vi "TEST_ASIC_MAJ_(3RD)_NEW.vi"(4 "Voltages comprobation":dbl[](array[numeric])=[0.05, 0.1, 0.2, 0.5, 0.8], 7 "Serial number":string="SN_023", 8 "error in":errorcluster, 9 "Cycles Burst":i32=10000, 10 "Channels":i32[](array[numeric])=[0, 1, 2, 3, 4, 5, 6], 11 "Instrument VISA in":T1={"AWG VISA"="generadorpulsos", "Oscilloscope  VISA "="Oscilloscope", "Integration Board IP"="172.16.7.43", "connection ID"=refnum, "report out"=refnum, "report file path"=path "C:/Documents and Settings/CTA_LAB01/Desktop/L0_Asic/L0 Asic Test Data"}) -> (0 "error out":errorcluster, 3 "Instrument VISA out":T1={"AWG VISA"="generadorpulsos", "Oscilloscope  VISA "="Oscilloscope", "Integration Board IP"="172.16.7.43", "connection ID"=refnum, "report out"=refnum, "report file path"=path "C:/Documents and Settings/CTA_LAB01/Desktop/L0_Asic/L0 Asic Test Data"}, 5 "ThresholdOut":i32[][](array[numeric])=[[519, 514, 509, 509, 509, 514, 519], [523, 518, 513, 513, 513, 518, 523], [527, 522, 517, 517, 517, 522, 527], [531, 526, 521, 516, 521, 526, 531], [535, 530, 525, 520, 525, 530, 535]])   [LabVIEW 2012]
uses:
  <vilib>/Utility/NIReport.llb/NI_report.lvclass
  <vilib>/Utility/NIReport.llb/HTML/NI_HTML.lvclass
  Sum_Abrilader/L0_Sum_Adder Folder/C/Program Files/National Instruments/LabVIEW 2012/instr.lib/Agilent 81150/Agilent 81150.lvlib
  <instrlib>/Agilent 8000 Series/Agilent 8000 Series.lvlib
panel:
  out "VmeasuredOut":dbl=0.024730000000000002 format="%.2f"
  in  "Threshold Limits":i32[](array[numeric])=[512, 1024]
  in  "Attenuation":i32[](array[numeric])=[15]
  out "read buffer 4":string="-1.1794E-08;2.150E-09;9.99999E+37;2.170E-09;1.310E-02;1.163E-02\n"
  out "report file path":path=path "C:/Documents and Settings/CTA_LAB01/Desktop/L0_Asic/L0 Asic Test Data"
  in  "time to wait":dbl=10.0
  out "Data output":dbl[][](array[numeric])
  out "read buffer 3":string
  out "appended array":dbl[](array[numeric])=[0.024730000000000002, 0.0, 2.17e-09, 0.0, 9.99999e+37, 0.0, 2.15e-09, 0.0, -1.1794e-08, 0.0, 0.0]
  out "points quantity":dbl
  out "Numeric":i32=2147483647
  in  "Save NOW!":bool
  in  "End 2":bool=TRUE
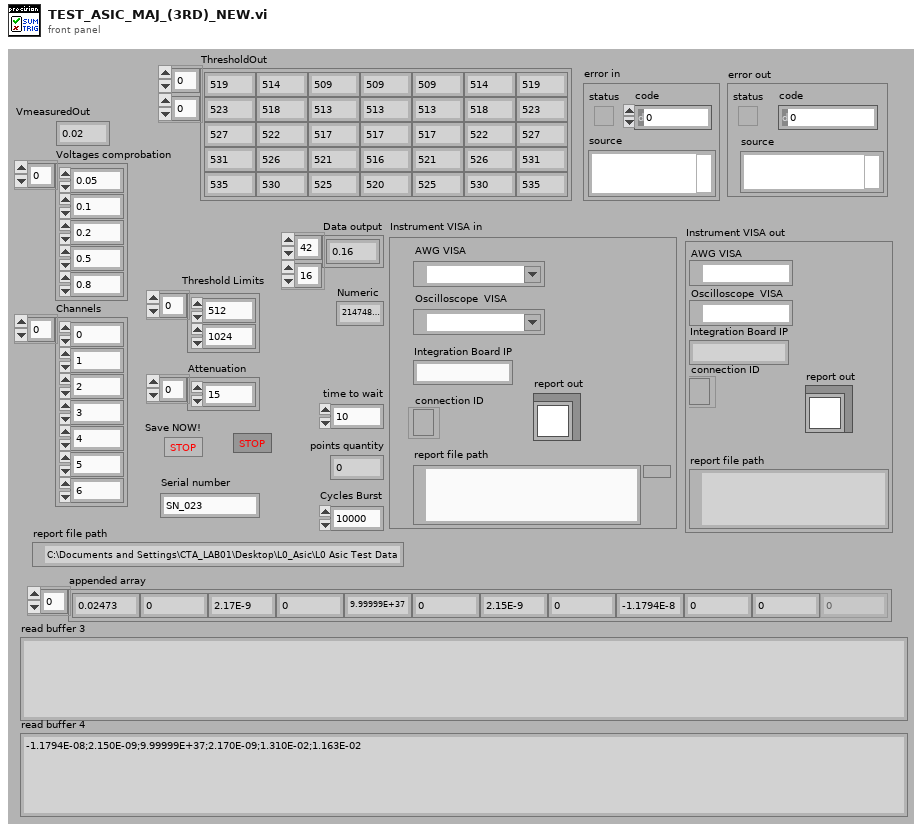
[diagram p1: front panel]
types:
  T1 = cluster{"AWG VISA":refnum<visa-resource-name>, "Oscilloscope  VISA ":refnum<visa-resource-name>, "Integration Board IP":string, "connection ID":refnum<k5>, "report out":refnum<class "NI_report.lvclass">, "report file path":path}
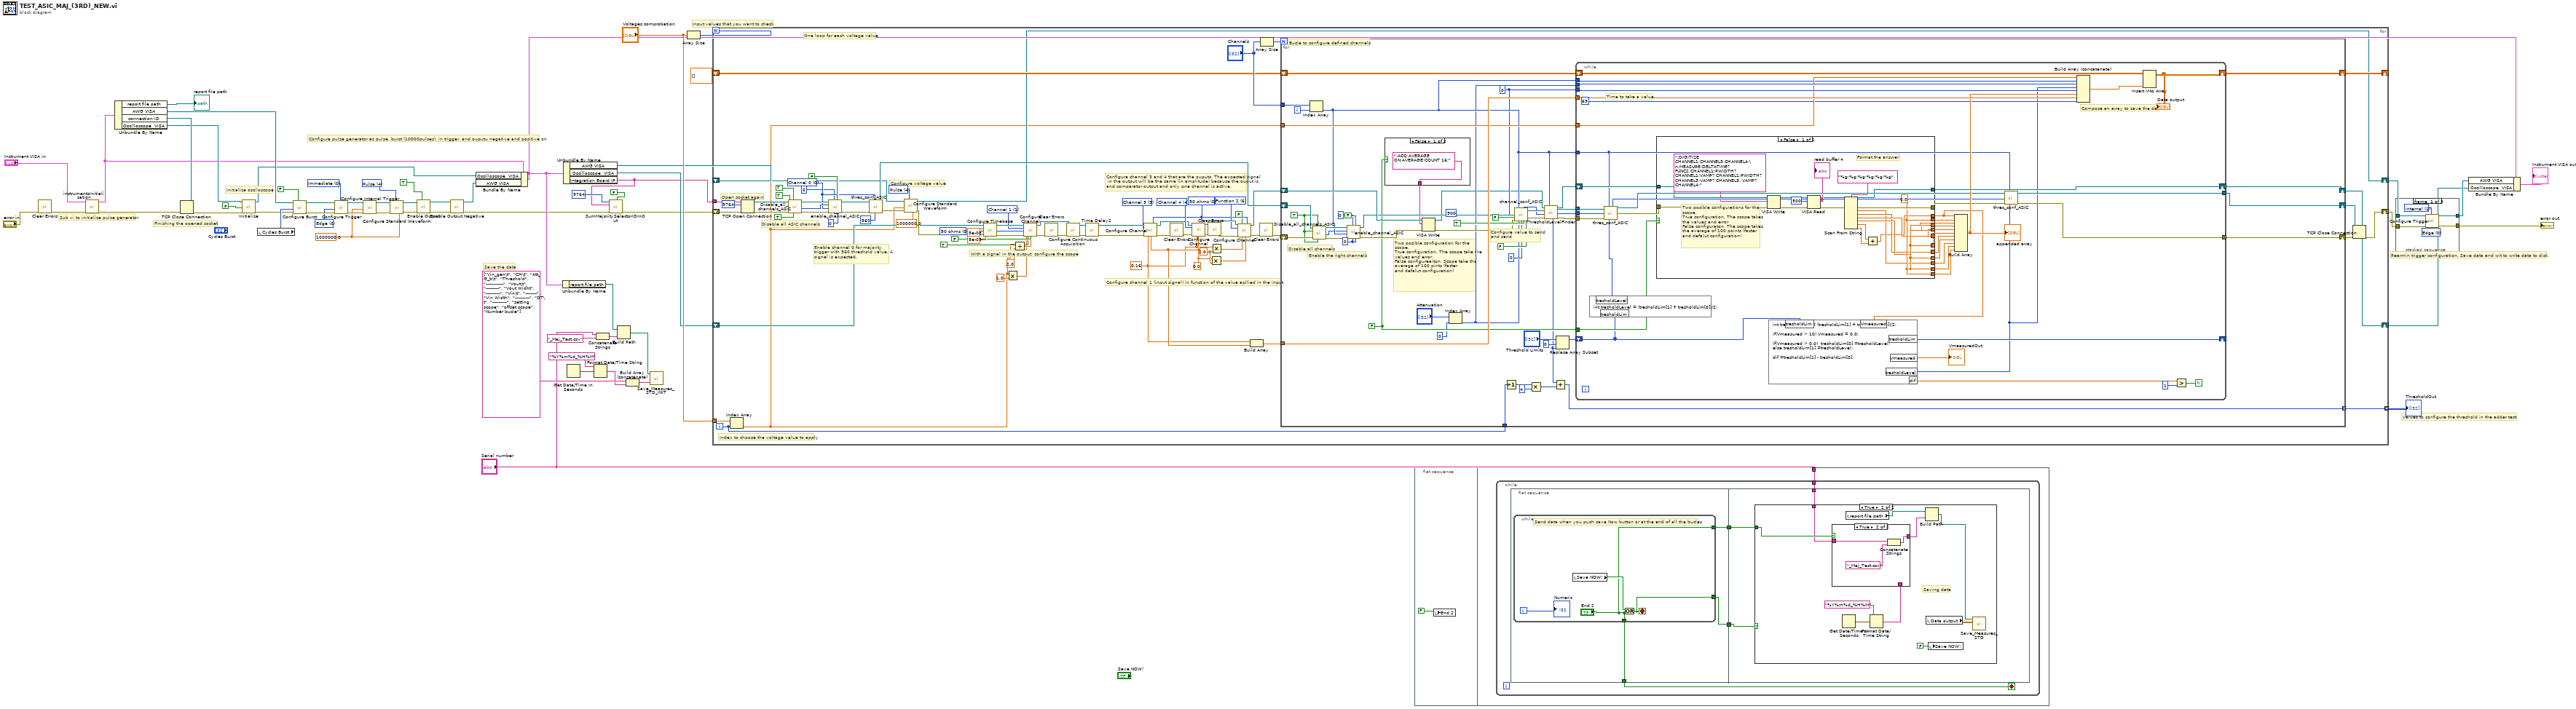
[diagram p0: block diagram]
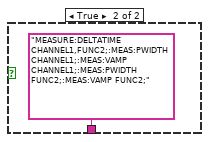
[diagram p2: hidden frame]
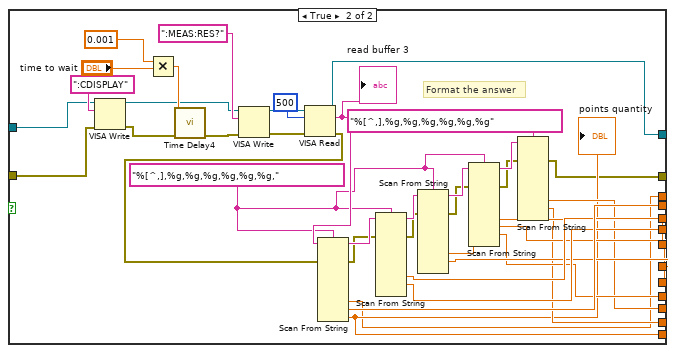
[diagram p3: hidden frame]
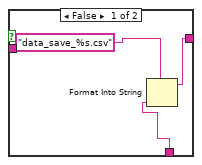
[diagram p5: hidden frame]
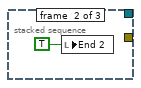
[diagram p6: hidden frame]
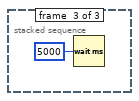
[diagram p7: hidden frame]
diagram:
  w25 = 1000000.0 ("Frequency (1000.0 Hz)")
  w50 = u16 0 items=["Immediate", "Internal", "External", "Software Trigger Function"] ("Trigger Source (0: Immediate)")
  w51 = u16 0 items=["Edge", "Level"] ("Trigger Mode (0: Edge)")
  w55 = u16 4 items=["Sine", "Square", "Ramp Up", "Ramp Down", "Pulse", "Noise", "DC"] ("Waveform (0: Sine)")
  # "Values to configure the threshold in the adder test."
  # "Save the data"
  # "Rearmin trigger configuration. Save data and wit to write data to disk."
  # "Input values that you want to check"
  # "Configure pulse generator as pulse, burst (10000pulses), in trigger, and ouputu negative and positive on"
  # "Initialize osciloscope"
  # "Finishing the opened socket"
  # "Sub vi to initialize pulse generator"
  n1 = call <vilib>:"Clear Errors.vi"("error in (no error)"="error in") -> ("error out"=w57:errorcluster)  [unwired: 6 in]
  n2 = call "instrumentsInitialization.vi"("error in"=w57, "Instrument VISA in"="Instrument VISA in") -> ("error out"=w44:errorcluster, "Instrument VISA out"=w35:T1)  [unwired: 8 in]
  n3 = Unbundle By Name(w35) -> ("report file path"=→"report file path":path, "AWG VISA"=w40:refnum<visa-resource-name>, "connection ID"=w45:refnum<k5>, "Oscilloscope  VISA"=w41:refnum<visa-resource-name>)
  n4 = TCP Close Connection(connection ID=w45, error in (no error)=w44) -> (error out=w39:errorcluster)  [unwired: 1 in, 1 out]
  n5 = call <instrlib>:"Initialize.vi"("error in (no error)"=w39, "Reset (True)"=FALSE ("ID Query (True)"), "VISA resource name"=w41) -> ("error out"=w21:errorcluster, "VISA resource name out"=w38:refnum<visa-resource-name>)  [unwired: 7 in]
  n6 = local read "Cycles Burst"() -> (w54:i32)
  n7 = call <instrlib>:"Configure Burst.vi"("Enable Burst (F: Disable)"=FALSE, "error in (no error)"=w21, "Burst Count (2)"=w54, "VISA resource name"=w40) -> ("error out"=w53:errorcluster, "VISA resource name out"=w52:refnum<visa-resource-name>)  [unwired: 6 in]
  n8 = call <instrlib>:"Configure Trigger.vi"("Trigger Source (0: Immediate)"=w50, "error in (no error)"=w53, "Trigger Mode (0: Edge)"=w51, "VISA resource name"=w52) -> ("error out"=w49:errorcluster, "VISA resource name out"=w48:refnum<visa-resource-name>)  [unwired: 6 in]
  n9 = call <instrlib>:"Configure Internal Trigger.vi"("error in (no error)"=w49, "Frequency (100000.0 Hz)"=w25, "VISA resource name"=w48) -> ("error out"=w46:errorcluster, "VISA resource name out"=w47:refnum<visa-resource-name>)  [unwired: 7 in]
  n10 = call <instrlib>:"Configure Standard Waveform.vi"("Frequency (1000.0 Hz)"=w25, "Waveform (0: Sine)"=w55, "error in (no error)"=w46, "VISA resource name"=w47) -> ("error out"=w37:errorcluster, "VISA resource name out"=w36:refnum<visa-resource-name>)  [unwired: 6 in]
  n11 = call <instrlib>:"Enable Output.vi"("Enable Output (T: Enable)"=TRUE, "error in (no error)"=w37, "VISA resource name"=w36) -> ("error out"=w24:errorcluster, "VISA resource name out"=w23:refnum<visa-resource-name>)  [unwired: 7 in]
  n12 = call "Enable Output Negative.vi"("error in (no error)"=w24, "VISA resource name"=w23) -> ("error out"=w5:errorcluster, "VISA resource name out"=w22:refnum<visa-resource-name>)  [unwired: 8 in]
  n13 = Bundle By Name(cluster=w35, "Oscilloscope  VISA"=w38, "AWG VISA"=w22) -> (w8:T1)
  n14 = Unbundle By Name(w8) -> ("report file path"=w9:path)
  n15 = Unbundle By Name(w8) -> ("AWG VISA"=w19:refnum<visa-resource-name>, "Oscilloscope  VISA"=w20:refnum<visa-resource-name>, "Integration Board IP"=w3:string)
  n16 = Get Date/Time In Seconds() -> (seconds since 1Jan1904=w14:timestamp)
  n17 = Format Date/Time String(time format string (%c)="%Y%m%d_%H%M", seconds (now)=w14) -> (date/time string=w12:string)  [unwired: 1 in]
  n18 = Concatenate Strings("Serial number", "_Maj_Test.csv" ("format string")) -> (w10:string)
  n19 = call "SumMajoritySelectorIDInOut.vi"("On Sum\nOff Majority"=FALSE, "error in"=w5, "address"=w3, "remote port or service name"=u16 9764) -> ("error out"=w6:errorcluster)  [unwired: 7 in]
  n20 = Build Path(base path=w9, name or relative path=w10) -> (appended path=w17:path)
  n21 = Build Array (concatenate)(string[] ["Vin_gen\t", "CH\t", "Att_G_b\t", "Threshold", "------------", "Vout\t", "---------", "Vout Widht", "----------", "Vin\t", "--------", "Vin Width", "----------", "DT\t", "----------", "setting scope", "offset scope", "Number bucle"] ("appended array"), w12) -> (w15:string[])
  n22 = call "Save_Measures_STD_INIT.vi"("appended array"=w15, "file path (dialog if empty)"=w17) -> ()  [unwired: 10 in]
  n23 = Array Size(array="Voltages comprobation") -> (size(s)=w29:i32)
  n24 = for {
    N: w29 -> [_]
    tunnel: w3 -> [w134]
    tunnel: "Voltages comprobation" -> [w133]
    shift-right: [w94] -> _
    shift-left: dbl[][] [] -> [w95]
    shift-right: [w75] -> w27
    shift-left: w20 -> [w71]
    shift-right: [w135] -> w32
    shift-left: w6 -> [w72]
    shift-right: [w70] -> w26
    shift-left: w19 -> [w64]
    tunnel: [w61] -> w1 mode=indexing
    i -> [w60]
    w63 = 0.16 ("Vertical Range (2.0 V)")
    w76 = 0.0 ("Vertical Offset (0.0 V)")
    w93 = u32 0 ("Clip_sel_b")
    w101 = 2.0 ("y")
    w78 = u32 0 items=["50 ohms", "1 Mohms"] ("Input Impedance (1: 1 Mohms)")
    w86 = u16 0 items=["Channel 0", "Channel 1", "Channel 2", "Channel 3", "Channel 4", "Channel 5", "Channel 6"] ("Channel")
    w121 = u32 0 items=["50 ohms", "1 Mohms"] ("Input Impedance (1: 1 Mohms)")
    w124 = 1 items=["Channel 1"=1, "Channel 2"=2, "Channel 3"=3, "Channel 4"=4] ("Channel (1: Channel 1)")
    w105 = u16 6 items=["Function 1"=5, "Function 2"=6, "Function 3"=7, "Function 4"=8] ("Math Channel (5: Function 1)")
    w77 = 3 items=["Channel 1"=1, "Channel 2"=2, "Channel 3"=3, "Channel 4"=4] ("Channel (1: Channel 1)")
    w119 = 4 items=["Channel 1"=1, "Channel 2"=2, "Channel 3"=3, "Channel 4"=4] ("Channel (1: Channel 1)")
    w131 = u16 4 items=["Sine", "Square", "Ramp Up", "Ramp Down", "Pulse", "Noise", "DC"] ("Waveform (0: Sine)")
    # "Configure channel 3 and 4 that are the ouputs. The expected signal\n in the output will be the same (in amplitude) because the ouput is and comparator output and only one channel is active."
    # "Configure channel 1 (input signal) in function of the value apllied in the input"
    # "With a signal in the output, configure the scope"
    # "Enable channel 0 for majority trigger with 560 threshold value. A signal is expected."
    # "Disable all ASIC channels"
    # "Open socket again"
    # "Configure voltage value"
    # "Index to choose the voltage value to apply"
    # "One loop for each voltage value"
    n25 = Index Array(array=w133, index=w60) -> (element=w62:dbl)
    n26 = TCP Open Connection(address=w134, remote port or service name=u16 9764, error in (no error)=w72) -> (connection ID=w115:refnum<k5>, error out=w114:errorcluster)  [unwired: 2 in]
    n27 = call "Disable_all_channels_ASIC.vi"("CompBuf_en_b"=TRUE, "Att_en_b"=TRUE, "error in"=w114, "Clip_en_b"=TRUE, "connection ID"=w115) -> ("error out"=w113:errorcluster, "id_out"=w111:i32, "connection ID out"=w112:refnum<k5>)  [unwired: 4 in]
    n28 = call "enable_channel_ASIC.vi"("Clip_sel_b"=w93, "maj/sum"=FALSE, "Ib_clipVb"=w93, "Att gain"=u32 0, "error in"=w113, "Channel"=w86, "id_in"=w111, "connection ID"=w112) -> ("error out"=w89:errorcluster, "connection ID out"=w91:refnum<k5>)  [unwired: 1 in, 1 out]
    n29 = call "thres_conf_ASIC.vi"("threshold"=u32 560, "Ring"=w86, "error out 3"=w89, "connection ID"=w91) -> ("error out 2"=w88:errorcluster, "connection ID out"=w90:refnum<k5>)  [unwired: 4 in, 2 out]
    n30 = call <instrlib>:"Configure Standard Waveform.vi"("Frequency (1000.0 Hz)"=1000000.0, "Waveform (0: Sine)"=w131, "error in (no error)"=w88, "Amplitude (1.0 Vpp)"=w62, "VISA resource name"=w64) -> ("error out"=w128:errorcluster, "VISA resource name out"=w70:refnum<visa-resource-name>)  [unwired: 5 in]
    n31 = call <instrlib>:"Configure Timebase.vi"("error in (no error)"=w128, "Position (0.0 s)"=8e-09, "Timebase (0.005 s)"=5e-08, "VISA resource name"=w71) -> ("error out"=w125:errorcluster, "VISA resource name out"=w126:refnum<visa-resource-name>)  [unwired: 6 in]
    n32 = Multiply(x=w62, y=1.0) -> (x*y=w102:dbl)
    n33 = Divide(x=w62, y=2.0) -> (x/y=w110:dbl)
    n34 = call <instrlib>:"Configure Channel.vi"("VISA resource name"=w126, "Enable Channel (Enable)"=TRUE, "BW Limit 20MHz (Disable)"=FALSE, "Input Impedance (1: 1 Mohms)"=w121, "Channel (1: Channel 1)"=w124, "error in (no error)"=w125, "Vertical Range (2.0 V)"=w102, "Vertical Offset (0.0 V)"=w110) -> ("VISA resource name out"=w67:refnum<visa-resource-name>, "error out"=w123:errorcluster)  [unwired: 6 in]
    n35 = call <vilib>:"Clear Errors.vi"("error in (no error)"=w123) -> ("error out"=w66:errorcluster)  [unwired: 6 in]
    n36 = call <instrlib>:"Configure Continuous Acquisition.vi"("error in (no error)"=w66, "VISA resource name"=w67) -> ("error out"=w104:errorcluster, "VISA resource name out"=w79:refnum<visa-resource-name>)  [unwired: 8 in]
    n37 = call "Time Delay2"("error in (no error)"=w104) -> ("error out"=w80:errorcluster)  [unwired: 10 in]
    n38 = call <instrlib>:"Configure Channel.vi"("VISA resource name"=w79, "Input Impedance (1: 1 Mohms)"=w78, "Channel (1: Channel 1)"=w77, "error in (no error)"=w80, "Vertical Range (2.0 V)"=w63, "Vertical Offset (0.0 V)"=w76) -> ("VISA resource name out"=w81:refnum<visa-resource-name>, "error out"=w82:errorcluster)  [unwired: 8 in]
    n39 = call <vilib>:"Clear Errors.vi"("error in (no error)"=w82) -> ("error out"=w116:errorcluster)  [unwired: 6 in]
    n40 = call <instrlib>:"Configure Channel.vi"("VISA resource name"=w81, "Input Impedance (1: 1 Mohms)"=w78, "Channel (1: Channel 1)"=w119, "error in (no error)"=w116, "Vertical Range (2.0 V)"=w63, "Vertical Offset (0.0 V)"=w76) -> ("VISA resource name out"=w107:refnum<visa-resource-name>, "error out"=w117:errorcluster)  [unwired: 8 in]
    n41 = call <vilib>:"Clear Errors.vi"("error in (no error)"=w117) -> ("error out"=w108:errorcluster)  [unwired: 6 in]
    n42 = Multiply(x=w76, y=w101) -> (x*y=w100:dbl)
    n43 = Multiply(x=w63, y=w101) -> (x*y=w106:dbl)
    n44 = call <instrlib>:"Configure Channel.vi"("VISA resource name"=w107, "Enable Channel (Enable)"=FALSE, "Input Impedance (1: 1 Mohms)"=w78, "Channel (1: Channel 1)"=w105, "error in (no error)"=w108, "Vertical Range (2.0 V)"=w106, "Vertical Offset (0.0 V)"=w100) -> ("VISA resource name out"=w74:refnum<visa-resource-name>, "error out"=w109:errorcluster)  [unwired: 7 in]
    n45 = Build Array(w63, w76) -> (w98:dbl[])
    n46 = call <vilib>:"Clear Errors.vi"("error in (no error)"=w109) -> ("error out"=w99:errorcluster)  [unwired: 6 in]
    n47 = Array Size(array="Channels") -> (size(s)=w97:i32)
    n48 = for {
      N: w97 -> [_]
      tunnel: w98 -> [w184]
      tunnel: "Channels" -> [w183]
      shift-right: [w185] -> w94
      shift-left: w95 -> [w181]
      tunnel: w62 -> [w180]
      shift-right: [w179] -> w75
      shift-left: w74 -> [w178]
      shift-right: [w177] -> w73
      shift-left: w99 -> [w174]
      shift-right: [w176] -> w69
      shift-left: w90 -> [w171]
      tunnel: [w163] -> w61 mode=indexing
      tunnel: w60 -> [w162]
      i -> [w182]
      w154 = FALSE
      (unwired) u32 500 ("byte count")
      w157 = u32 0 ("Ib_ClipVb")
      w168 = u32 0 ("Ib_clipVb")
      w169 = TRUE ("Att_en_b")
      # "Configure value to send and send"
      # "Two posible configuration for the scope. \nTrue configuration. The scope take the values and error\nFalse configureaiton. Scope take the average of 100 pints (faster\nand defalut configuration)"
      # "Enable the right channels"
      # "Disable all channels"
      # "Bucle to configure defined channels"
      n49 = Index Array(array=w183, index=w182) -> (element=w166:i32)
      n50 = call "Disable_all_channels_ASIC.vi"("CompBuf_en_b"=w169, "Att_en_b"=w169, "error in"=w174, "Clip_en_b"=w169, "connection ID"=w171) -> ("error out"=w175:errorcluster, "id_out"=w165:i32, "connection ID out"=w172:refnum<k5>)  [unwired: 4 in]
      n51 = call "enable_channel_ASIC.vi"("Clip_sel_b"=w168, "maj/sum"=FALSE, "Ib_clipVb"=w168, "Att gain"=u32 0, "error in"=w175, "Channel"=w166, "id_in"=w165, "connection ID"=w172) -> ("error out"=w173:errorcluster, "connection ID out"=w170:refnum<k5>)  [unwired: 1 in, 1 out]
      n52 = case shown="False" w154 {
        tunnel: [":ACQ:AVERAGE ON;AVERAGE:COUNT 16;" ("write buffer") "MEASURE:DELTATIME CHANNEL1,FUNC2;:MEAS:PWIDTH CHANNEL1;:MEAS:VAMP CHANNEL1;:MEAS:PWIDTH FUNC2;:MEAS:VAMP FUNC2;" ("write buffer")] -> w156
        frame False {
        }
        frame True {
        }
      }
      n53 = VISA Write(VISA resource name=w178, write buffer=w156, error in (no error)=w173) -> (VISA resource name out=w146:refnum<visa-resource-name>, error out=w155:errorcluster)  [unwired: 1 out]
      n54 = Index Array(array="Attenuation", index=u32 0 ("Ib_ClipVb")) -> (element=w153:i32)
      n55 = Increment(x=w162) -> (x+1=w140:i32)
      n56 = call "channel_conf_ASIC.vi"("connection ID"=w170, "Ring"=w166, "Clip_sel_b"=w157, "CompBuf_en_b"=FALSE, "error out"=w155, "Att gain"=w153, "Ib_ClipVb"=u32 0, "Clip_en_b"=TRUE, "Att_en_b"=FALSE) -> ("Id out"=w145:i32, "connection ID out"=w150:refnum<k5>, "error out 2"=w152:errorcluster)  [unwired: 2 in, 2 out]
      n57 = Multiply(x=w140, y=4) -> (x*y=w138:i32)
      n58 = call "ThresholdLevelFinder.vi"("Channel"=w166, "error in (no error)"=w152, "id_in"=w145, "connection ID"=w150, "VISA resource name"=w146) -> ("error out"=w151:errorcluster, "id_out"=w149:i32, "connection ID out"=w148:refnum<k5>, "VISA resource name out"=w147:refnum<visa-resource-name>, "threshold out"=w139:i32)  [unwired: 2 in]
      n59 = Add(x=w139, y=w138) -> (x+y=w163:i32)
      n60 = Replace Array Subset(array="Threshold Limits", new element=w139, index=u32 0 ("Att gain")) -> (w143:i32[])
      n61 = while {
        tunnel: w184 -> [w227]
        tunnel: [w198] -> w177
        tunnel: w151 -> [w192]
        tunnel: w157 -> [w212]
        tunnel: w166 -> [w207]
        tunnel: w153 -> [w211]
        tunnel: w166 -> [w188]
        tunnel: w149 -> [w194]
        tunnel: w180 -> [w209]
        shift-right: [w226] -> w179
        shift-left: w147 -> [w213]
        shift-right: [w223] -> w185
        shift-left: w181 -> [w228]
        tunnel: w154 -> [w208]
        shift-right: [w203] -> _
        shift-left: w143 -> [w190]
        tunnel: w148 -> [w195]
        tunnel: [w210] -> w176
        stop <- w200 continue-if-true
        # "Compose an array to save the data"
        # "Time to take a value"
        n62 = formula code="int tresholdLevel = (tresholdLim[1] + tresholdLim[0])/2;"("tresholdLim"=w190) -> ("tresholdLevel"=w189:i32)
        n63 = call "thres_conf_ASIC.vi"("threshold"=w189, "Ring"=w188, "error out 3"=w192, "Id in"=w194, "connection ID"=w195) -> ("error out 2"=w191:errorcluster, "connection ID out"=w196:refnum<k5>, "Id out"=w193:i32)  [unwired: 3 in, 1 out]
        n64 = case shown="False" w208 {
          tunnel: [w243 w277] -> w226
          tunnel: [w241 w276] -> w225
          tunnel: [w237 w269] -> w222
          tunnel: [w241 w268] -> w221
          tunnel: [w238 w267] -> w220
          tunnel: [w241 w266] -> w219
          tunnel: [w236 w265] -> w218
          tunnel: [w241 w264] -> w217
          tunnel: [w235 w263] -> w216
          tunnel: [w241 w262] -> w215
          tunnel: [w241 w261] -> w214
          tunnel: [w242 w259] -> w199
          tunnel: w213 -> [w244 w252]
          tunnel: [w231 w250] -> w197
          tunnel: w191 -> [w230 w249]
          frame False {
            w241 = 0.0 ("points quantity")
            # "Format the answer"
            # "Two posible configurations for the scope. \nTrue configuration. The scope takes the values and error\nFalse configuraton. The scope takes the average of 100 points (faster\nand defalut configuration)"
            n65 = VISA Write(VISA resource name=w244, write buffer=":DIGITIZE CHANNEL1,CHANNEL3,CHANNEL4;\n:MEASURE:DELTATIME? FUNC2,CHANNEL1;PWIDTH? CHANNEL1;VAMP? CHANNEL1;PWIDTH? CHANNEL3;VAMP? CHANNEL3; VAMP? CHANNEL4;", error in (no error)=w230) -> (VISA resource name out=w239:refnum<visa-resource-name>, error out=w240:errorcluster)  [unwired: 1 out]
            n66 = VISA Read(VISA resource name=w239, byte count=u32 500, error in (no error)=w240) -> (VISA resource name out=w243:refnum<visa-resource-name>, read buffer=w247:string, error out=w245:errorcluster)  [unwired: 1 out]
            "read buffer 4" <- w247
            n67 = Scan From String(format string="%g;%g;%g;%g;%g;%g", input string=w247, error in=w245) -> (error out=w242:errorcluster, output 1=w235:dbl, output 2=w236:dbl, output 3=w238:dbl, output 4=w237:dbl, output 5=w233:dbl, output 6=w232:dbl)  [unwired: 7 in, 2 out]
            n68 = Add(x=w233, y=w232) -> (x+y=w231:dbl)
          }
          frame True {
            w271 = "%[^,],%g,%g,%g,%g,%g,%g," ("format string")
            # "Format the answer"
            n69 = VISA Write(VISA resource name=w252, write buffer=":CDISPLAY", error in (no error)=w249) -> (VISA resource name out=w254:refnum<visa-resource-name>, error out=w251:errorcluster)  [unwired: 1 out]
            n70 = Multiply(x=0.001, y="time to wait") -> (x*y=w279:dbl)
            n71 = call "Time Delay4"("error in (no error)"=w251, "Delay Time (s)"=w279) -> ("error out"=w278:errorcluster)  [unwired: 9 in]
            n72 = VISA Write(VISA resource name=w254, write buffer=":MEAS:RES?", error in (no error)=w278) -> (VISA resource name out=w286:refnum<visa-resource-name>, error out=w285:errorcluster)  [unwired: 1 out]
            n73 = VISA Read(VISA resource name=w286, byte count=u32 500, error in (no error)=w285) -> (VISA resource name out=w277:refnum<visa-resource-name>, read buffer=w282:string, error out=w260:errorcluster)  [unwired: 1 out]
            "read buffer 3" <- w282
            n74 = Scan From String(format string=w271, input string=w282, error in=w260) -> (remaining string=w275:string, error out=w255:errorcluster, output 5=w250:dbl, output 6=w276:dbl, output 7=w261:dbl)  [unwired: 12 in, 1 out]
            "points quantity" <- w261
            n75 = Scan From String(format string=w271, input string=w275, error in=w255) -> (remaining string=w272:string, error out=w256:errorcluster, output 5=w269:dbl, output 6=w268:dbl)  [unwired: 13 in, 1 out]
            n76 = Scan From String(format string=w271, input string=w272, error in=w256) -> (remaining string=w273:string, error out=w257:errorcluster, output 5=w267:dbl, output 6=w266:dbl)  [unwired: 13 in, 1 out]
            n77 = Scan From String(format string=w271, input string=w273, error in=w257) -> (remaining string=w274:string, error out=w258:errorcluster, output 5=w265:dbl, output 6=w264:dbl)  [unwired: 13 in, 1 out]
            n78 = Scan From String(format string="%[^,],%g,%g,%g,%g,%g,%g", input string=w274, error in=w258) -> (error out=w259:errorcluster, output 5=w263:dbl, output 6=w262:dbl)  [unwired: 13 in, 2 out]
          }
        }
        n79 = formula code="int tresholdLevel = (tresholdLim[1] + tresholdLim[0])/2;\n\nif(Vmeasured > 10) Vmeasured = 0.0;\n\nif(Vmeasured > 0.0)  tresholdLim[0] =tresholdLevel;\nelse tresholdLim[1] =tresholdLevel;\n\ndif =tresholdLim[1] - tresholdLim[0];"("Vmeasured"=w197, "tresholdLim"=w190) -> ("dif"=w205:dbl, "tresholdLevel"=w201:i32, "tresholdLim"=w203:i32[], "Vmeasured"=→"VmeasuredOut":dbl)
        n80 = Build Array(w197, w225, w222, w221, w220, w219, w218, w217, w216, w215, w214) -> (w224:dbl[])
        "appended array" <- w224
        n81 = call "thres_conf_ASIC.vi"("threshold"=w201, "Ring"=w188, "error out 3"=w199, "Id in"=w193, "connection ID"=w196) -> ("error out 2"=w198:errorcluster, "connection ID out"=w210:refnum<k5>)  [unwired: 3 in, 2 out]
        n82 = Build Array (concatenate)(w209, w207, w211, w201, w212, w224, w227, 69) -> (w229:dbl[])
        n83 = Insert Into Array(array=w228, new element=w229) -> (w223:dbl[][])  [unwired: 2 in]
        "Data output" <- w223
        n84 = Greater?(x=w205, y=1) -> (0:w200:bool)
      }
    }
    n85 = TCP Close Connection(connection ID=w69, error in (no error)=w73) -> (error out=w135:errorcluster)  [unwired: 1 in, 1 out]
  }
  "ThresholdOut" <- w1
  n86 = flat-sequence {
    tunnel: "Serial number" -> [w288]
    frame #0 {
      n87 = local write "End 2"(FALSE ("End")) -> ()
    }
    frame #1 {
      n88 = while {
        tunnel: w288 -> [w289]
        stop <- w290 stop-if-true
        n89 = flat-sequence {
          tunnel: [w295] -> w292
          tunnel: [w294] -> w291
          tunnel: [w293] -> w290
          tunnel: w292 -> [w302]
          tunnel: w291 -> [w301]
          tunnel: w289 -> [w300]
          frame #0 {
            n90 = while {
              tunnel: [w298] -> w295
              tunnel: ["End 2"] -> w294
              tunnel: ["End 2"] -> w293
              i -> [w297]
              stop <- w298 stop-if-true
              # "Send data when you push save Now button or at the end of all the bucles"
              n91 = local read "Save NOW!"() -> (w299:bool)
              n92 = Or(x=w299, y="End 2") -> (x .or. y?=w298:bool)
              "Numeric" <- w297
            }
          }
          frame #1 {
            n93 = case shown="True" w302 {
              tunnel: w301 -> [_ w309]
              tunnel: w300 -> [_ w303]
              frame False {
              }
              frame True {
                # "Saving data"
                n94 = Get Date/Time In Seconds() -> (seconds since 1Jan1904=w307:timestamp)
                n95 = local read "report file path"() -> (w311:path)
                n96 = Format Date/Time String(time format string (%c)="%Y%m%d_%H%M", seconds (now)=w307) -> (date/time string=w305:string)  [unwired: 1 in]
                n97 = case shown="True" w309 {
                  tunnel: [w314 w318] -> w308
                  tunnel: w305 -> [w313 _]
                  tunnel: w303 -> [_ w316]
                  frame False {
                    n98 = Format Into String(format string="data_save_%s.csv", w313) -> (resulting string=w314:string)  [unwired: 2 in, 1 out]
                  }
                  frame True {
                    n99 = Concatenate Strings(w316, "_Maj_Test.csv" ("format string")) -> (w318:string)
                  }
                }
                n100 = Build Path(base path=w311, name or relative path=w308) -> (appended path=w312:path)
                n101 = local read "Data output"() -> (w304:dbl[][])
                n102 = local write "Save NOW!"(FALSE ("Save NOW!")) -> ()
                n103 = call "Save_Measures_STD.vi"("Data in"=w304, "file path (dialog if empty)"=w312) -> ()  [unwired: 10 in]
              }
            }
          }
        }
      }
    }
  }
  n104 = stacked-sequence {
    tunnel: w32 -> [w322 _ _]
    tunnel: [w321 _ _] -> w18
    tunnel: w26 -> [w320 _ _]
    tunnel: [w319 _ _] -> w28
    frame #0 {
      w323 = u16 1 items=["Immediate", "Internal", "External", "Software Trigger Function"] ("Trigger Source (0: Immediate)")
      w324 = u16 0 items=["Edge", "Level"] ("Trigger Mode (0: Edge)")
      n105 = call <instrlib>:"Configure Trigger.vi"("Trigger Source (0: Immediate)"=w323, "error in (no error)"=w322, "Trigger Mode (0: Edge)"=w324, "VISA resource name"=w320) -> ("error out"=w321:errorcluster, "VISA resource name out"=w319:refnum<visa-resource-name>)  [unwired: 6 in]
    }
    frame #1 {
      n106 = local write "End 2"(TRUE ("End 2")) -> ()
    }
    frame #2 {
      n107 = Wait (ms)(milliseconds to wait=u32 5000) -> ()  [unwired: 1 out]
    }
  }
  "error out" <- w18
  n108 = Bundle By Name(cluster=w8, "AWG VISA"=w28, "Oscilloscope  VISA"=w27) -> (→"Instrument VISA out":T1)
